vi "模字量AD输入统计结果.vi"   [LabVIEW 2010]
uses:
  全局量/自动测试结果.vi
  全局量/试验配置信息.vi
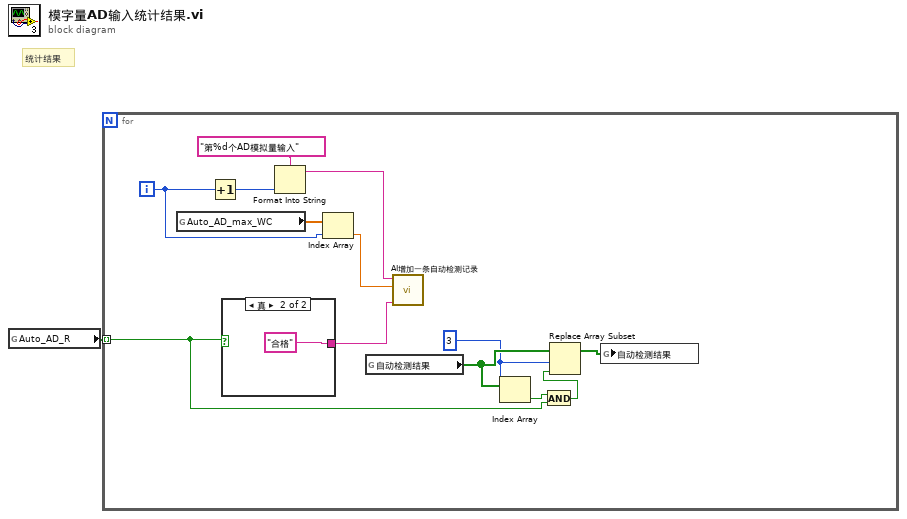
[diagram p0: block diagram]
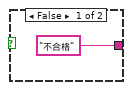
[diagram p2: hidden frame]
diagram:
  # "统计结果"
  n1 = global read "自动测试结果.vi" "Auto_AD_R"() -> (w1:bool[])
  n2 = for {
    tunnel: w1 -> [w2] mode=indexing
    i -> [w9]
    w5 = 3 ("索引")
    n3 = global read "自动测试结果.vi" "Auto_AD_max_WC"() -> (w10:dbl[])
    n4 = Increment(x=w9) -> (x+1=w14:i32)
    n5 = case shown="真" w2 {
      tunnel: ["不合格" "合格"] -> w11
      frame False {
      }
      frame True {
      }
    }
    n6 = Format Into String(format string="第%d个AD模拟量输入", w14) -> (resulting string=w12:string)  [unwired: 2 in, 1 out]
    n7 = Index Array(array=w10, index=w9) -> (element=w8:dbl)
    n8 = global read "试验配置信息.vi" "自动检测结果"() -> (w6:bool[])
    n9 = call "AI增加一条自动检测记录.vi"("测试结果"=w11, "最大误差"=w8, "测试内容"=w12) -> ()  [unwired: 9 in]
    n10 = Index Array(array=w6, index=w5) -> (element=w4:bool)
    n11 = And(x=w4, y=w2) -> (x .and. y?=w3:bool)
    n12 = Replace Array Subset(array=w6, new element=w3, index=w5) -> (w7:bool[])
    n13 = global write "试验配置信息.vi" "自动检测结果"(w7) -> ()
  }
